vi "Create Polynomial From Roots (DBL).vi"(11 "Roots":dbl[](array[numeric]) format="%#.6g") -> (0 "error":i32, 3 "P(x)":dbl[](array[numeric]) format="%#.6g")   [LabVIEW 2017, in "NI_AALPro.lvlib"]
doc: "Creates polynomial <B>P(x)</B> from its roots. Wire data to the <B>Roots</B> input to determine the polymorphic instance to use or manually select the instance."
uses:
  NI_AALPro.lvlib
  Multiply Polynomials (DBL).vi
  Leja Order Roots (DBL).vi
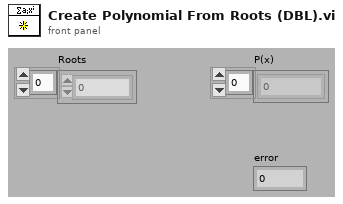
[diagram p1: front panel]
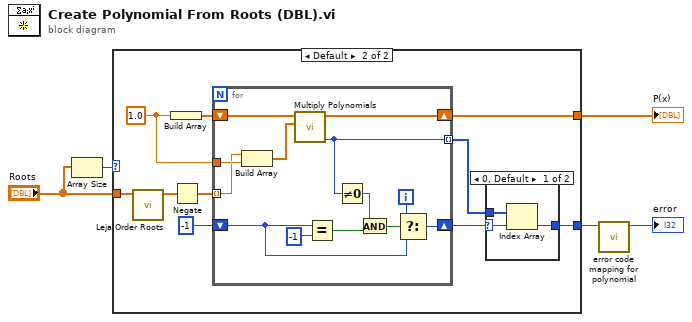
[diagram p0: block diagram]
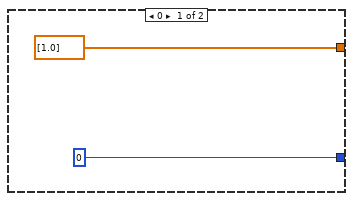
[diagram p2: hidden frame]
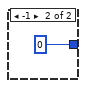
[diagram p3: hidden frame]
diagram:
  n1 = Array Size(array="Roots") -> (size(s)=w4:i32)
  n2 = case shown="Default" w4 {
    tunnel: [dbl[] [1.0] ("BDL") w15] -> w5
    tunnel: "Roots" -> [_ w10]
    tunnel: [0 w11] -> w2
    frame 0 {
    }
    frame Default {
      w16 = 1.0
      n3 = call-poly "Leja Order Roots.vi"("Roots"=w10) -> ("Roots of Leja Order"=w9:dbl[])  [unwired: 10 in]
      n4 = Build Array(w16) -> (w17:dbl[])
      n5 = Negate(x=w9) -> (-x=w14:dbl[])
      n6 = for {
        shift-right: [w34] -> w15
        shift-left: w17 -> [w31]
        tunnel: w16 -> [w33]
        tunnel: w14 -> [w30] mode=indexing
        shift-right: [w24] -> w8
        shift-left: -1 -> [w22]
        tunnel: [w28] -> w12 mode=indexing
        i -> [w23]
        n7 = Build Array(w30, w33) -> (w32:dbl[])
        n8 = call-poly "Multiply Polynomials.vi"("Q(x)"=w32, "P(x)"=w31) -> ("error"=w28:i32, "P(x)*Q(x)"=w34:dbl[])  [unwired: 8 in]
        n9 = Equal?(x=w22, y=-1) -> (x = y?=w25:bool)
        n10 = Not Equal To 0?(x=w28) -> (x != 0?=w29:bool)
        n11 = And(x=w29, y=w25) -> (x .and. y?=w27:bool)
        n12 = Select(t=w23, s=w27, f=w22) -> (s? t:f=w24:i32)
      }
      n13 = case shown="0, Default" w8 {
        selector: w8 -> [w18 _]
        tunnel: w12 -> [w20 _]
        tunnel: [w19 0 ("error")] -> w11
        frame 0, Default {
          n14 = Index Array(array=w20, index=w18) -> (element=w19:i32)
        }
        frame -1 {
        }
      }
    }
  }
  "P(x)" <- w5
  n15 = call "error code mapping for polynomial.vi"("error in"=w2) -> ("error out"=→"error":i32)  [unwired: 10 in]
